vi "Benchmark.vi"() -> ()   [LabVIEW 2018]
doc: "_Test_"
panel:
  in  "Tag Lookup":enum32{"By Name", "By Ref"}(radio)=enum."By Ref"
  out "Values":dbl[](array[numeric])
  out "Avg Read Time (s)":dbl format="%0.9f"
  out "Avg Write Time (s)":dbl format="%0.9f"
  out "Avg Creation Time (s)":dbl format="%0.9f"
  in  "#Tags":i32=100000
  # "Tested at 100000 tags"
  # "Tag Engine: 0.000018355"
  # "VIRegisters: 0.000865646"
  # "Tag Engine: 0.000001485"
  # "VIRegisters: 0.000904695"
  # "Tag Engine: 0.000001384"
  # "VIRegisters: 0.000879308"
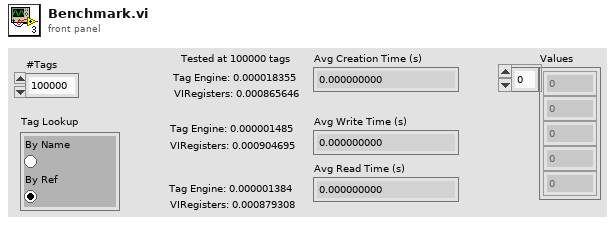
[diagram p1: front panel]
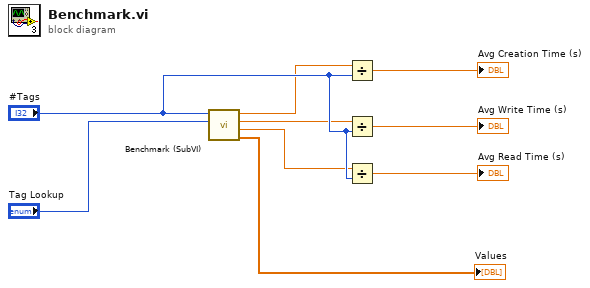
[diagram p0: block diagram]
diagram:
  n1 = call "Benchmark (SubVI).vi"("Tag Lookup"="Tag Lookup", "#Tags"="#Tags") -> ("Values"=→"Values":dbl[], "Read Time"=w2:dbl, "Write Time"=w3:dbl, "Creation Time"=w4:dbl)  [unwired: 6 in]
  n2 = Divide(x=w4, y="#Tags") -> (x/y=→"Avg Creation Time (s)":dbl)
  n3 = Divide(x=w3, y="#Tags") -> (x/y=→"Avg Write Time (s)":dbl)
  n4 = Divide(x=w2, y="#Tags") -> (x/y=→"Avg Read Time (s)":dbl)
